vi "Test_Status.vi"(11 "Status In":T1[](array[typedef])=[enum."Not Ready to Switch On", enum."Switch On Disabled", enum."Ready to Switch On", enum."Switched On", enum."Operation enable", enum."Quick Stop Active", enum."Fault Reaction Active", enum."Fault"]) -> (1 "Pass?":bool[](array[boolean]), 2 "Word":u16[](array[numeric]) format="%08b", 3 "Status Out":T1[](array[typedef]))   [LabVIEW 2017, in "WordManipulationTests.lvlib"]
uses:
  WordManipulationTests.lvlib
  Utilities/StateMachine.ctl
  Utilities/WordManipulationLibrary.lvlib
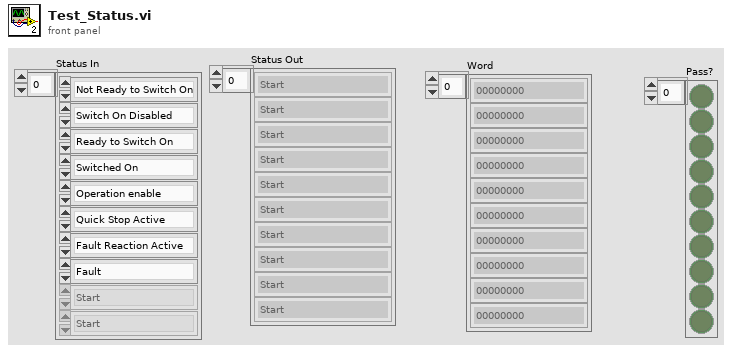
[diagram p1: front panel]
types:
  T1 = typedef "WordManipulationLibrary.lvlib/StateMachine.ctl" = enum16{"Start", "Not Ready to Switch On", "Switch On Disabled", "Ready to Switch On", "Switched On", "Operation enable", "Quick Stop Active", "Fault Reaction Active", "Fault"}
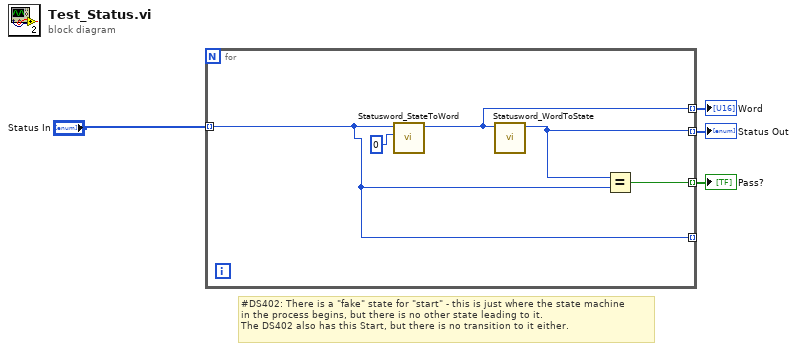
[diagram p0: block diagram]
diagram:
  # "#DS402: There is a \"fake\" state for \"start\" - this is just where the state machine\nin the process begins, but there is no other state leading to it.\nThe DS402 also has this Start, but there is no transition to it either."
  n1 = for {
    tunnel: [w5] -> w4 mode=indexing
    tunnel: [w8] -> w2 mode=indexing
    tunnel: [w6] -> _ mode=indexing
    tunnel: [w7] -> w3 mode=indexing
    tunnel: "Status In" -> [w6] mode=indexing
    n2 = call "Statusword_StateToWord.vi"("StatusWord In"=u16 0 ("ControlWord In"), "CurrentStatus"=w6) -> ("StatusWord Out"=w7:u16)  [unwired: 9 in]
    n3 = call "Statusword_WordToState.vi"("Data_In"=w7) -> ("Status"=w8:T1)  [unwired: 10 in]
    n4 = Equal?(x=w8, y=w6) -> (x = y?=w5:bool)
  }
  "Pass?" <- w4
  "Word" <- w3
  "Status Out" <- w2
